vi "PAN_Shutdown.vi"(7 "cmdQ":refnum<queue>, 9 "Modules":string[](array[string])=["GUNSC", "GFITS", "LOGIC", "BUFMGR"]) -> ()   [LabVIEW 2016]
uses:
  PAN_cmdStruct.ctl
panel:
  in  "cmd struct":T1
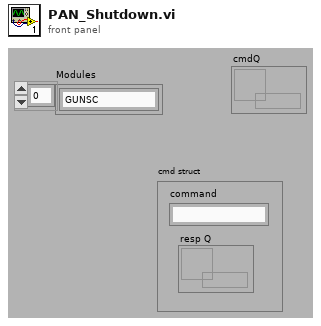
[diagram p1: front panel]
types:
  T1 = typedef "PAN_cmdStruct.ctl" = cluster{"command":string, "resp Q":refnum<queue>}
  T2 = enum16{"add", "delete", "clean", "shutdown", "hold", "continue", "modify"}
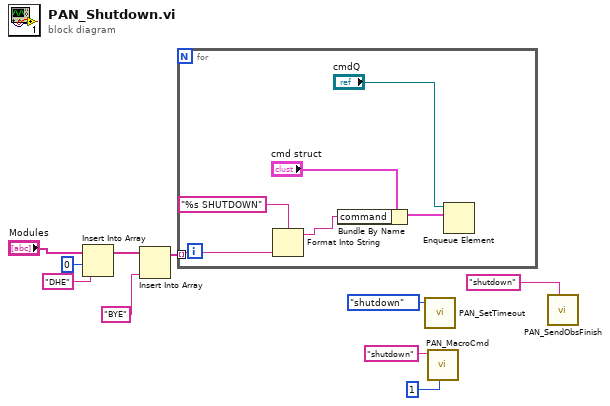
[diagram p0: block diagram]
diagram:
  n1 = Insert Into Array(array="Modules", index=0, new element="DHE" ("new element/subarray")) -> (w6:string[])
  n2 = Insert Into Array(array=w6, new element="BYE" ("new element/subarray")) -> (w4:string[])  [unwired: 1 in]
  n3 = for {
    tunnel: w4 -> [w13] mode=indexing
    n4 = Format Into String(format string="%s SHUTDOWN", w13) -> (resulting string=w11:string)  [unwired: 2 in, 1 out]
    n5 = Bundle By Name(cluster="cmd struct", "command"=w11) -> (w15:T1)
    n6 = Enqueue Element(queue="cmdQ", element=w15) -> ()  [unwired: 1 in, 4 out]
  }
  n7 = call "PAN_SetTimeout.vi"("action"=T2."shutdown") -> ()  [unwired: 3 in, 8 out]
  n8 = call "PAN_MacroCmd.vi"("timeout in ms (-1)"=1, "Command"="shutdown") -> ()  [unwired: 1 in, 9 out]
  n9 = call "PAN_SendObsFinish.vi"("command"="shutdown" ("obsID")) -> ()  [unwired: 3 in, 8 out]
